vi "Query Sequencer ARB File Duration.vi"(8 "error in (no error)":errorcluster, 9 "Index (0)":i32, 10 "Instance (1)":i32=1, 11 "VISA resource name":refnum<visa-resource-name>) -> (0 "error out":errorcluster, 2 "Duration":dbl format="%^.3e", 3 "VISA resource name out":refnum<visa-resource-name>)   [LabVIEW 2020, in "Rohde&Schwarz CMXP GPRF.lvlib"]
doc: "Queries the duration of the ARB file with the specified Index.\n\nAttribute:\n-\n\nRemote-control command:\nSOURce:GPRF:GEN<i>:SEQuencer:APOol:DURation?"
uses:
  <instrlib>/Rohde&Schwarz CMXP GPRF/Rohde&Schwarz CMXP GPRF.lvlib
  <instrlib>/Rohde&Schwarz CMXP GPRF/Private/rsidr_core.llb/rsidr_core.lvlib
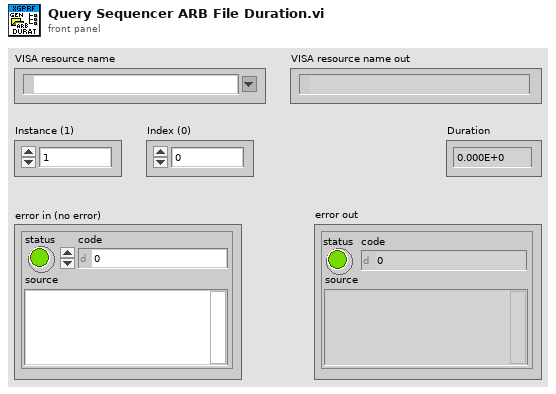
[diagram p1: front panel]
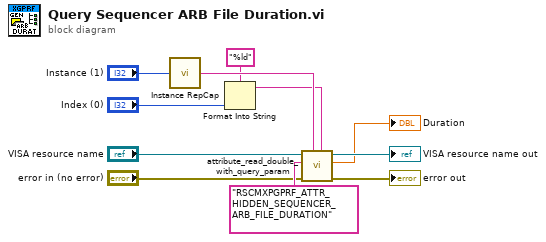
[diagram p0: block diagram]
diagram:
  n1 = call <instrlib>:"Instance RepCap.vi"("Instance in"="Instance (1)") -> ("Instance out"=w11:string)
  n2 = Format Into String(format string="%ld", "Index (0)") -> (resulting string=w8:string)  [unwired: 2 in, 1 out]
  n3 = call <instrlib>:"attribute_read_double_with_query_param.vi"("Query Parameter (None)"=w8, "Repeated Capability (\"\")"=w11, "error in"="error in (no error)", "Attribute ID"="RSCMXPGPRF_ATTR_HIDDEN_SEQUENCER_ARB_FILE_DURATION", "VISA resource name"="VISA resource name") -> ("error out"=→"error out":errorcluster, "Double out"=→"Duration":dbl, "VISA resource name out"=→"VISA resource name out":refnum<visa-resource-name>)  [unwired: 4 in]
